vi "Run.vi"(8 "error in (no error)":errorcluster, 9 "s on last turn":dbl, 10 "Maze (0: Empty, -1: Enemy. >0: Teammate":i32[][](array[numeric]), 11 "Expand in":refnum<class "Expand.lvclass">) -> (0 "error out":errorcluster, 1 "Direction":T1, 2 "Action":T2, 3 "Expand out":refnum<class "Expand.lvclass">, 4 "Replicated":refnum<class "Runner.lvclass">)   [LabVIEW 2014, in "Expand.lvclass"]
uses:
  Expand.lvclass
  Action Enum.ctl
  SquareBattle.lvclass
  Runner.lvclass
  Direction Enum.ctl
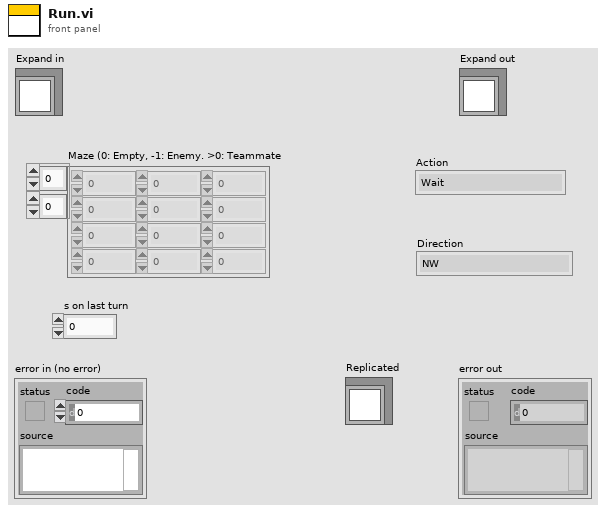
[diagram p1: front panel]
types:
  T1 = typedef "SquareBattle.lvclass/Direction Enum.ctl" = enum16{"NW", "N", "NE", "E", "SE", "S", "SW", "W"}
  T2 = typedef "SquareBattle.lvclass/Action Enum.ctl" = enum16{"Wait", "Move", "Attack", "Replicate"}
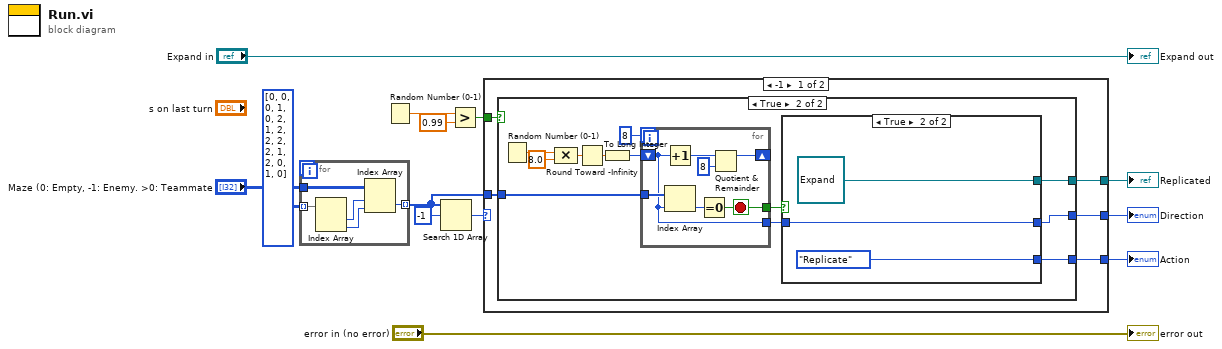
[diagram p0: block diagram]
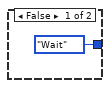
[diagram p2: hidden frame]
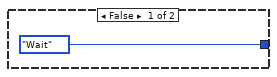
[diagram p3: hidden frame]
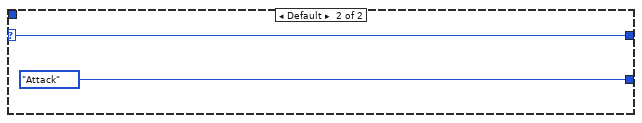
[diagram p4: hidden frame]
diagram:
  n1 = for {
    tunnel: "Maze (0: Empty, -1: Enemy. >0: Teammate" -> [w18]
    tunnel: i32[][] [[0, 0], [0, 1], [0, 2], [1, 2], [2, 2], [2, 1], [2, 0], [1, 0]] -> [w17] mode=indexing
    tunnel: [w14] -> w6 mode=indexing
    n2 = Index Array(array=w17) -> (element #1=w16:i32, element #2=w15:i32)  [unwired: 2 in]
    n3 = Index Array(array=w18, index (row)=w16, index (col)=w15) -> (element=w14:i32)
  }
  n4 = Random Number (0-1)() -> (number: 0 to 1=w3:dbl)
  n5 = Search 1D Array(1D array=w6, element=-1) -> (index of element=w9:i32)  [unwired: 1 in]
  n6 = Greater?(x=w3, y=0.99) -> (0:w2:bool)
  n7 = case shown="-1" w9 {
    selector: w9 -> [_ w49]
    tunnel: [w21 w49] -> w8
    tunnel: [w22 Action_Enum."Attack" ("Action")] -> w7
    tunnel: w6 -> [w23 _]
    tunnel: [w20 _] -> w5
    tunnel: w2 -> [w19 _]
    frame -1 {
      n8 = case shown="True" w19 {
        tunnel: w23 -> [_ w30]
        tunnel: [Action_Enum."Wait" ("Action") w28] -> w22
        tunnel: [_ w27] -> w21
        tunnel: [_ w25] -> w20
        frame False {
        }
        frame True {
          n9 = Random Number (0-1)() -> (number: 0 to 1=w35:dbl)
          n10 = Compound Arithmetic op=MULTIPLY(w35, 8.0 ("value")) -> (w33:dbl)
          n11 = Round Toward -Infinity(1:w33) -> (0:w32:dbl)
          n12 = To Long Integer(number=w32) -> (32bit integer=w31:i32)
          n13 = for {
            N: 8 -> [_]
            tunnel: w30 -> [w47]
            shift-right: [w43] -> _
            shift-left: w31 -> [w42]
            tunnel: [w42] -> w26
            tunnel: [w41] -> w29
            stop <- w41 stop-if-true
            n14 = Increment(x=w42) -> (x+1=w45:i32)
            n15 = Index Array(array=w47, index=w42) -> (element=w46:i32)
            n16 = Equal To 0?(x=w46) -> (x = 0?=w41:bool)
            n17 = Quotient & Remainder(x=w45, y=8) -> (x-y*floor(x/y)=w43:i32)  [unwired: 1 out]
          }
          n18 = case shown="True" w29 {
            tunnel: [Action_Enum."Wait" ("Action") Action_Enum."Replicate" ("Action")] -> w28
            tunnel: [_ w39] -> w27
            tunnel: w26 -> [_ w39]
            tunnel: [_ refnum<class "Expand.lvclass"> refnum ("Expand.lvclass")] -> w25
            frame False {
            }
            frame True {
            }
          }
        }
      }
    }
    frame Default {
    }
  }
  "Action" <- w7
  "Direction" <- w8
  "Replicated" <- w5
  "error out" <- "error in (no error)"
  "Expand out" <- "Expand in"
